vi "WriteStoreData.vi"(1 "Spots":T1[](array[typedef]) {"F2-Value overall" format="%.2f"; "tauerror" format="%.2f"; "Lifetime[ns]" format="%.2f"; "F2-Value TAC" format="%.2f"}, 2 "Enum":enum16{"Save", "Control"}(ring), 3 "Image Path":refnum<vi>) -> (0 "already x spots":i16)   [LabVIEW 2009]
uses:
  spotproperties.ctl
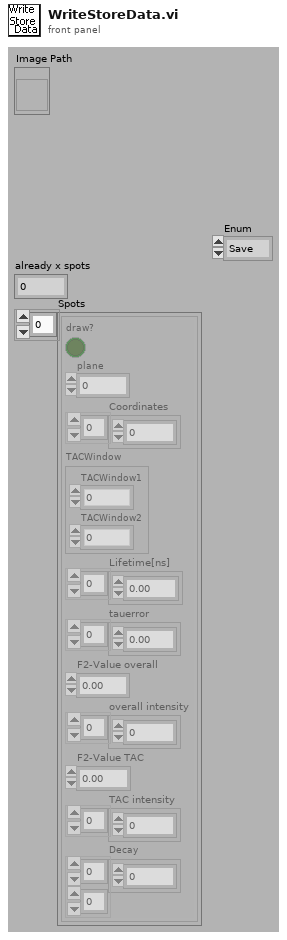
[diagram p1: front panel]
types:
  T1 = typedef "spotproperties.ctl" = cluster{"draw?":bool, "plane":u32, "Coordinates":i32[], "TACWindow":cluster{"TACWindow1":i32, "TACWindow2":i32}, "Lifetime[ns]":ext[], "tauerror":dbl[], "F2-Value overall":dbl, "overall intensity":u32[], "F2-Value TAC":dbl, "TAC intensity":u32[], "Decay":u32[][]}
  T2 = enum16{"Display", "change", "Get", "Set", "Set Ken"}
  T3 = enum16{"open", "open or create", "create or replace", "create", "open (read only)"}
  T4 = enum16{"read/write", "read-only", "write-only", "write-only (truncate)"}
  T5 = typedef "Settings.ctl" = cluster{"threshold":cluster{"max":u32, "min":u32}, "RGB or false color":bool, "16bit":bool, "log/lin axis":u16, "spotsize button":bool, "Pixelsize":u16, "autoscale x":bool, "autoscale y":bool, "correlation":bool, "ADC-Resolution":i32, "F2-lifetime":cluster{"display tau":bool, "display F2":bool, "Palette Number lifetime":enum32{"Gray", "Binary", "Gradient", "Rainbow", "Temperature"}, "Palette Number F2":enum32{"Gray", "Binary", "Gradient", "Rainbow", "Temperature"}, "max tau-Value":dbl, "min tau-Value":dbl, "max F2-Value":dbl, "min F2-Value":dbl}, "TAC-Window 1":u16, "TAC-Window 2":u16, "false color palette":cluster{"1":u32, "2":u32, "3":u32, "4":u32, "5":u32, "6":u32, "7":u32, "8":u32, "8 2":u32, "8 3":u32, "8 4":u32, "8 5":u32}, "rebinning":dbl}
  T6 = typedef "FIFOSettings_BH.ctt" = cluster{"Measurement":cluster{"Binning (ms)":sgl, "External Trigger Condition":u16, "Stop Condition:":u16, "Stop Count":dbl, "Buffer Size (Photons)":u16, "No of Channels":u16, "Ext Latch Delay":i16}, "ADC":cluster{"Module":u16, "ADC Resolution":i32, "Dither Range":i16, "Count Increment":i16, "Macro Time Clock":i16}, "SYNC":cluster{"SYNC ZC Level (mV)":sgl, "SYNC Freq Divider":i16, "SYNC Holdoff (ns)":sgl, "SYNC Threshold (mV)":sgl}, "TAC":cluster{"TAC Range (ns)":sgl, "TAC Gain":i16, "TAC Offset (%)":sgl, "TAC Limit Low (%)":sgl, "TAC Limit High (%)":sgl}, "CFD":cluster{"CFD Limit Low (mV)":sgl, "CFD Limit High (mV)":sgl, "CFD ZC Level (mV)":sgl, "CFD Holdoff (ns)":sgl}}
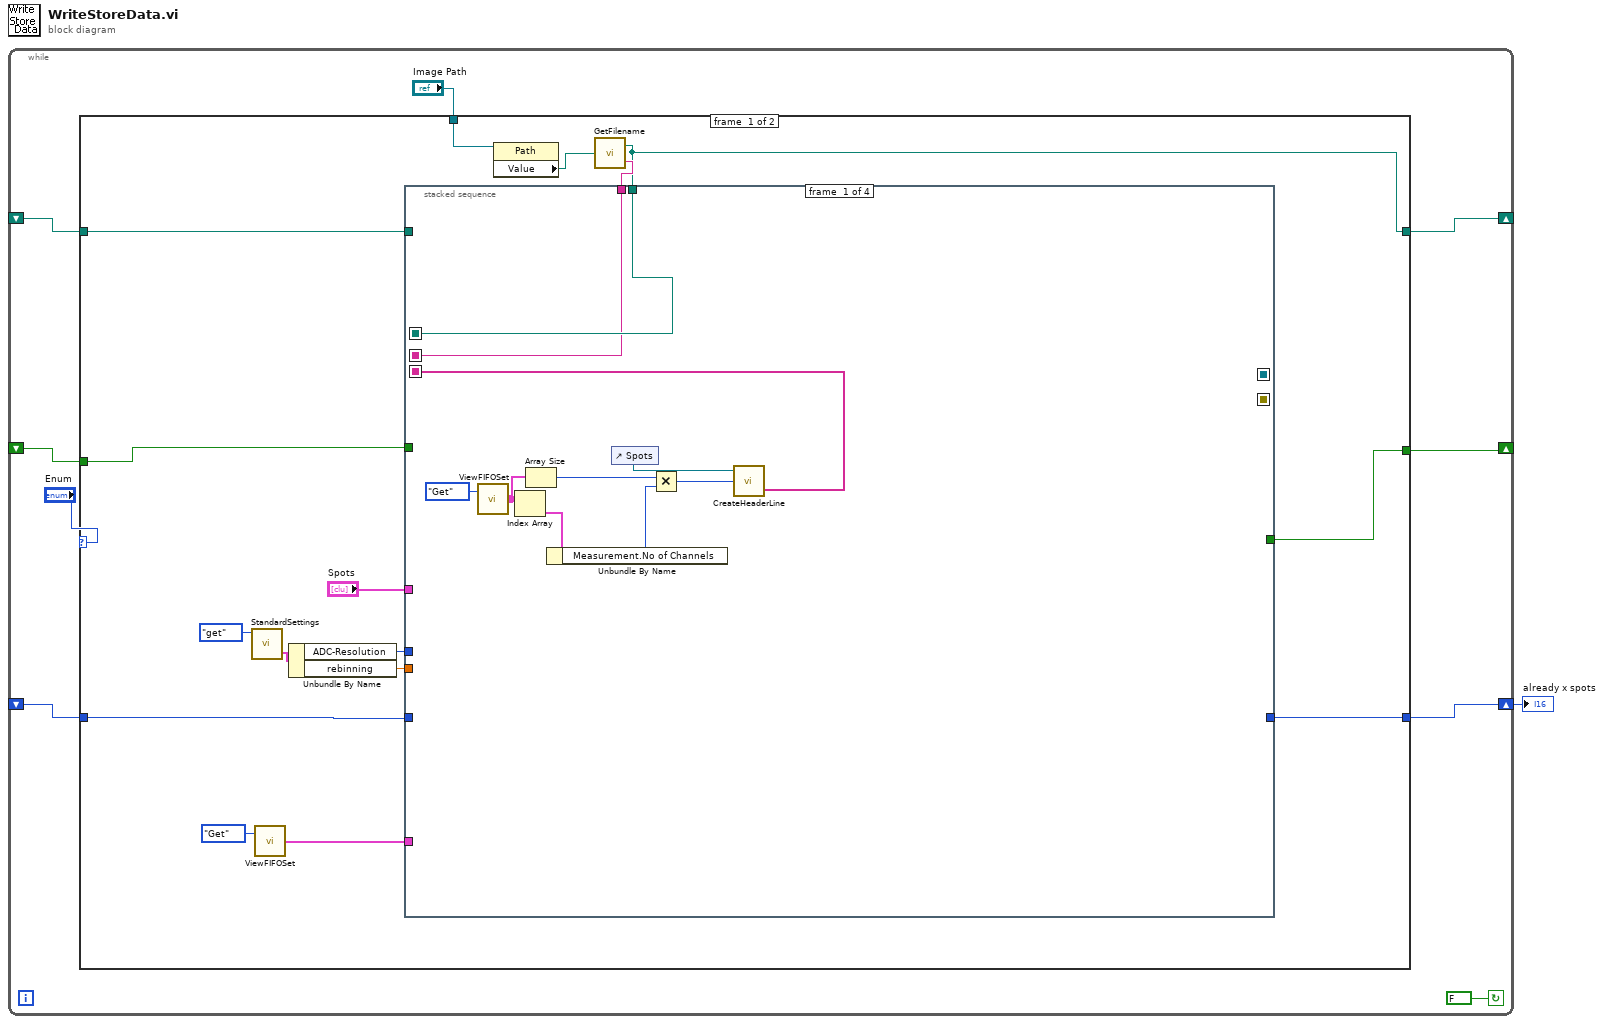
[diagram p0: block diagram]
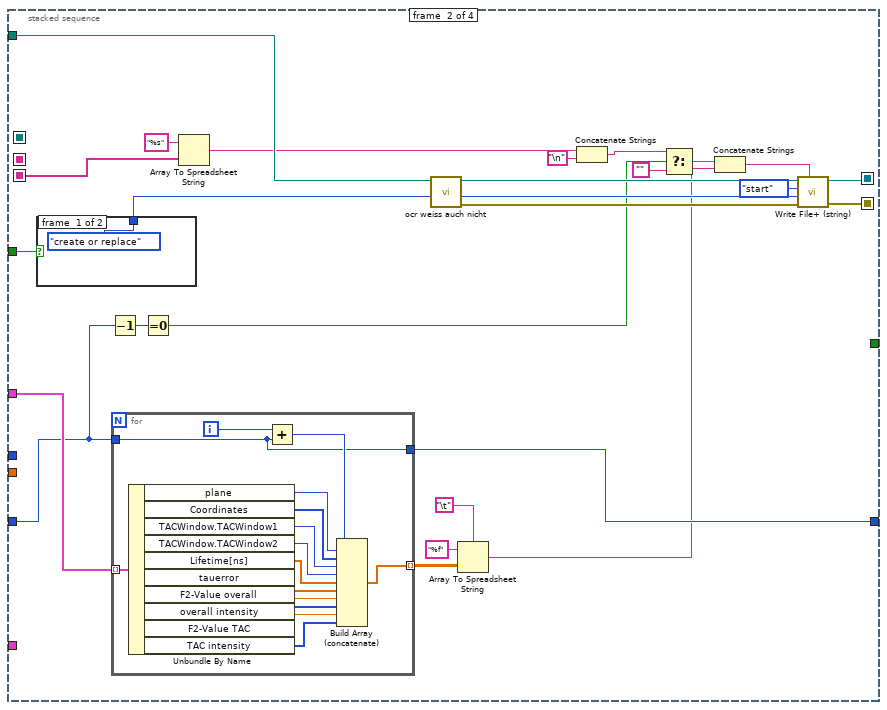
[diagram p2: hidden frame]
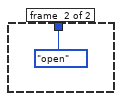
[diagram p3: hidden frame]
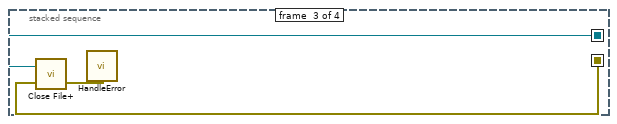
[diagram p4: hidden frame]
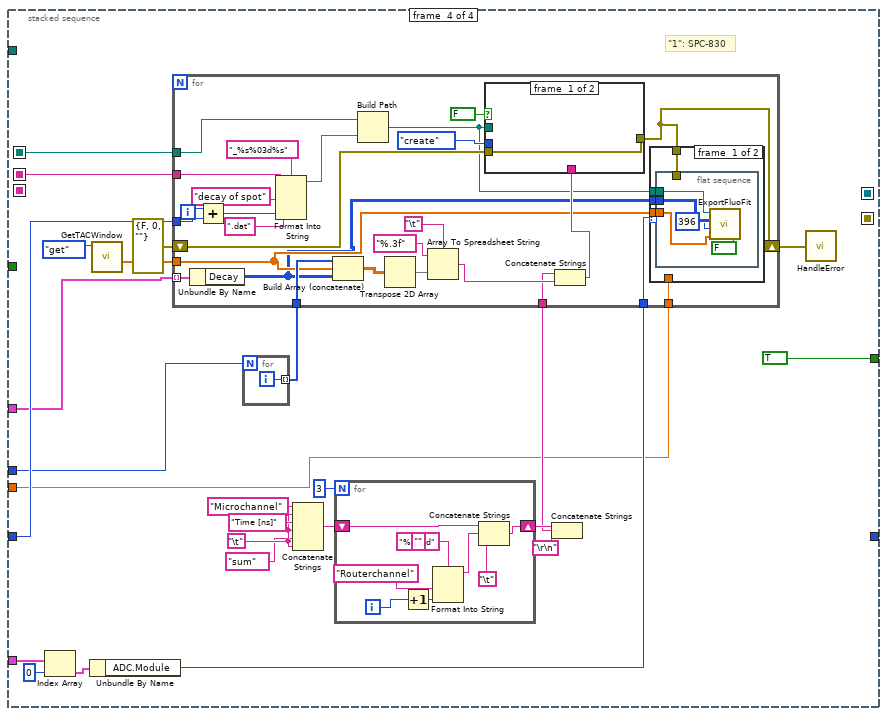
[diagram p5: hidden frame]
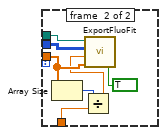
[diagram p6: hidden frame]
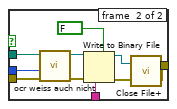
[diagram p7: hidden frame]
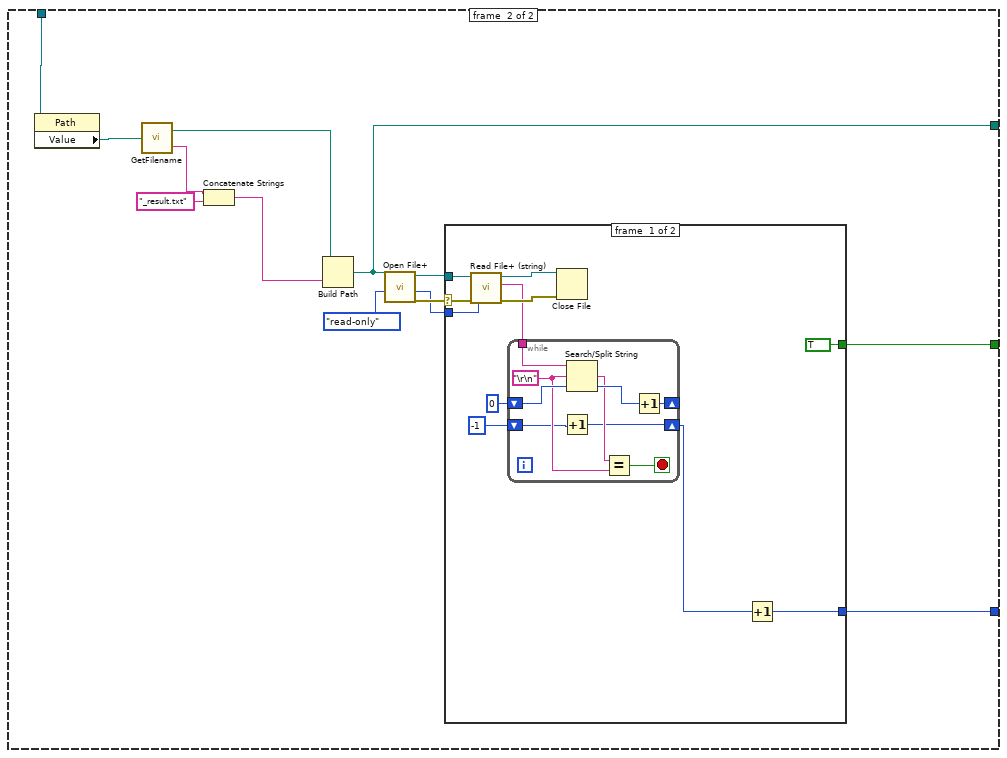
[diagram p8: hidden frame]
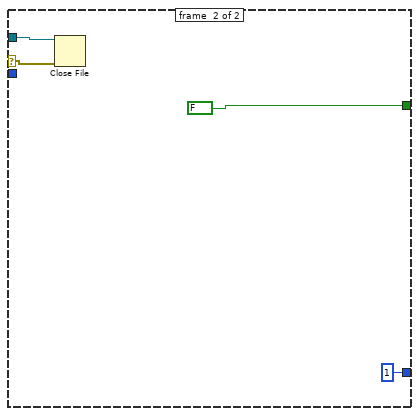
[diagram p9: hidden frame]
diagram:
  n1 = while {
    shift-right: [w8] -> _
    shift-left: _ -> [w7]
    shift-right: [w6] -> w1
    shift-left: _ -> [w5]
    shift-right: [w4] -> _
    shift-left: _ -> [w3]
    stop <- FALSE continue-if-true
    n2 = case shown="\"Save\", Default" "Enum" {
      tunnel: [w26 w183] -> w8
      tunnel: w7 -> [w25 _]
      tunnel: [w24 w171] -> w6
      tunnel: w5 -> [w18 _]
      tunnel: [w14 w173] -> w4
      tunnel: w3 -> [w23 _]
      tunnel: "Image Path" -> [w15 w172]
      frame #0 {
        n3 = call "StandardSettings.vi"("Enum"=enum16{"Load", "get", "Save", "set"}."get") -> ("StandardSettings"=w21:T5)  [unwired: 4 in]
        n4 = call "ViewFIFOSet.vi"("Enum"=T2."Get") -> ("FIFO Settings (Array)"=w12:T6[])  [unwired: 1 in]
        n5 = Unbundle By Name(w21) -> ("ADC-Resolution"=w20:i32, "rebinning"=w11:dbl)
        n6 = property class="Path"(reference=w15) -> ("Value"=w16:path)  [unwired: 1 in, 2 out]
        n7 = call "GetFilename.vi"("Value"=w16) -> ("base path"=w14:path, "name"=w17:string)
        n8 = stacked-sequence {
          seq-local: [w28 _ _ _] -> [_ _ _ w107]
          seq-local: [w27 _ _ _] -> [_ _ _ w95]
          seq-local: [w35 _ _ _] -> [_ w48 _ _]
          seq-local: [_ w61 _ _] -> [_ _ w82 _]
          seq-local: [_ w60 _ _] -> [_ _ w81 _]
          tunnel: "Spots" -> [_ w59 _ w92]
          tunnel: [_ _ _ TRUE] -> w26
          tunnel: w25 -> [_ w52 _ _]
          tunnel: [_ w51 _ _] -> w24
          tunnel: w18 -> [_ w44 _ w99]
          tunnel: w23 -> [_ w49 _ _]
          tunnel: w20 -> [_ _ _ w91]
          tunnel: w14 -> [w28 _ _ _]
          tunnel: w17 -> [w27 _ _ _]
          tunnel: w12 -> [_ _ _ w87]
          tunnel: w11 -> [_ _ _ w83]
          frame #0 {
            n9 = call "ViewFIFOSet.vi"("Enum"=T2."Get") -> ("FIFO Settings (Array)"=w30:T6[])  [unwired: 1 in]
            n10 = Index Array(array=w30) -> (element=w33:T6)  [unwired: 1 in]
            n11 = Array Size(array=w30) -> (size(s)=w31:i32)
            n12 = Unbundle By Name(w33) -> ("Measurement.No of Channels"=w32:u16)
            n13 = control-ref of="Spots"() -> (w36:refnum<vi>)
            n14 = Multiply(x=w31, y=w32) -> (x*y=w29:i32)
            n15 = call "CreateHeaderLine.vi"("No of channels"=w29, "Spots 3"=w36) -> ("Headline array"=w35:string[])  [unwired: 2 in]
          }
          frame #1 {
            n16 = case shown="True" w52 {
              tunnel: [T3."create or replace" ("function (open:0)") T3."open" ("function (open:0)")] -> w62
              frame #0 {
              }
              frame #1 {
              }
            }
            n17 = Decrement(x=w44) -> (x-1=w45:i16)
            n18 = for {
              tunnel: w59 -> [w79] mode=indexing
              tunnel: [w78] -> w58 mode=indexing
              tunnel: [w75] -> w51
              tunnel: w44 -> [w75]
              i -> [w77]
              n19 = Unbundle By Name(w79) -> ("plane"=w74:u32, "Coordinates"=w73:i32[], "TACWindow.TACWindow1"=w72:i32, "TACWindow.TACWindow2"=w71:i32, "Lifetime[ns]"=w70:ext[], "tauerror"=w69:dbl[], "F2-Value overall"=w68:dbl, "overall intensity"=w67:u32[], "F2-Value TAC"=w66:dbl, "TAC intensity"=w65:u32[])
              n20 = Add(x=w77, y=w75) -> (x+y=w76:i32)
              n21 = Build Array (concatenate)(w76, w74, w73, w72, w71, w70, w69, w68, w67, w66, w65) -> (w78:ext[])
            }
            n22 = Equal To 0?(x=w45) -> (x = 0?=w43:bool)
            n23 = Array To Spreadsheet String(array=w48, 3:"%s" ("format string")) -> (spreadsheet string=w46:string)  [unwired: 1 in]
            n24 = call "ocr weiss auch nicht.vi"("function (open:0)"=w62, "file path"=w49) -> ("error out"=w55:errorcluster, "file size (bytes)"=w53:i32, "refnum"=w56:refnum<file>)  [unwired: 6 in, 1 out]
            n25 = Array To Spreadsheet String(delimiter (Tab)="\t", array=w58, 3:"%f" ("format string")) -> (spreadsheet string=w39:string)
            n26 = Concatenate Strings(w46, "\n") -> (w42:string)
            n27 = Select(t=w42, s=w43, f="") -> (s? t:f=w40:string)
            n28 = Concatenate Strings(w40, w39) -> (w38:string)
            n29 = call "Write File+ (string).vi"("string"=w38, "error in (no error)"=w55, "pos offset (bytes:0)"=w53, "pos mode (rel. to end:1)"=enum16{"start", "end", "current"}."start", "refnum"=w56) -> ("error out"=w60:errorcluster, "dup refnum"=w61:refnum<file>)  [unwired: 2 in, 1 out]
          }
          frame #2 {
            n30 = call "Close File+.vi"("error in (no error)"=w81, "refnum"=w82) -> ("error out"=w80:errorcluster)  [unwired: 3 in, 2 out]
            n31 = call "HandleError.vi"("error in (no error)"=w80) -> ()
          }
          frame #3 {
            w94 = "\t"
            # "\"1\": SPC-830"
            n32 = Index Array(array=w87, index=0) -> (element=w85:T6)
            n33 = Unbundle By Name(w85) -> ("ADC.Module"=w84:u16)
            n34 = call "GetTACWindow.vi"("Enum"=enum16{"ini", "get", "quick"}."get") -> ("x-values"=w88:dbl[])  [unwired: 1 in, 8 out]
            n35 = for {
              N: w91 -> [_]
              tunnel: [w108] -> w97 mode=indexing
              i -> [w108]
            }
            n36 = Concatenate Strings("Microchannel" ("string"), w94, "Time [ns]" ("string"), w94, "sum" ("string"), w94) -> (w101:string)
            n37 = for {
              N: 3 -> [_]
              shift-right: [w116] -> w105
              shift-left: w101 -> [w115]
              i -> [w113]
              (unwired) "%s %d" ("format string")
              n38 = Increment(x=w113) -> (x+1=w112:i32)
              n39 = Format Into String(format string="", "Routerchannel", w112) -> (resulting string=w110:string)  [unwired: 2 in, 1 out]
              n40 = Concatenate Strings(w115, w110, "\t") -> (w116:string)
            }
            n41 = Concatenate Strings(w105, "\r\n") -> (w104:string)
            n42 = for {
              tunnel: w92 -> [w143] mode=indexing
              tunnel: w107 -> [w142]
              tunnel: w88 -> [w123]
              shift-right: [w121] -> w89
              shift-left: errorcluster {"status"=FALSE, "code"=0, "source"=""} ("error out") -> [w137]
              tunnel: w104 -> [w134]
              tunnel: w99 -> [w129]
              tunnel: w95 -> [w124]
              tunnel: w97 -> [w125]
              tunnel: w84 -> [w118]
              tunnel: w83 -> [w117]
              i -> [w130]
              n43 = Unbundle By Name(w143) -> ("Decay"=w119:u32[][])
              n44 = Add(x=w130, y=w129) -> (x+y=w128:i32)
              n45 = Format Into String(format string="_%s%03d%s", initial string=w124, "decay of spot", w128, ".dat" ("replace string (\"\")")) -> (resulting string=w132:string)  [unwired: 1 in, 1 out]
              n46 = Build Array (concatenate)(w125, w123, w119) -> (w140:dbl[][])
              n47 = Build Path(base path=w142, name or relative path=w132) -> (appended path=w122:path)
              n48 = Transpose 2D Array(2D array=w140) -> (transposed array=w139:dbl[][])
              n49 = Array To Spreadsheet String(delimiter (Tab)="\t", array=w139, 3:"%.3f" ("format string")) -> (spreadsheet string=w136:string)
              n50 = Concatenate Strings(w134, w136) -> (w135:string)
              n51 = case shown="False" FALSE {
                tunnel: w137 -> [w160 w166]
                tunnel: w135 -> [_ w165]
                tunnel: T3."create" ("function (open:0)") -> [_ w164]
                tunnel: w122 -> [_ w163]
                tunnel: [w160 w162] -> w121
                frame #0 {
                }
                frame #1 {
                  n52 = call "ocr weiss auch nicht.vi"("error in (no error)"=w166, "function (open:0)"=w164, "file path"=w163) -> ("error out"=w167:errorcluster, "refnum"=w168:refnum<file>)  [unwired: 5 in, 2 out]
                  n53 = Write to Binary File(file (use dialog)=w168, data=w165, error in=w167, 5:FALSE ("prepend array or string size? (T)")) -> (refnum out=w169:refnum<file>, error out=w170:errorcluster)  [unwired: 2 in, 1 out]
                  n54 = call "Close File+.vi"("error in (no error)"=w170, "refnum"=w169) -> ("error out"=w162:errorcluster)  [unwired: 3 in, 2 out]
                }
              }
              n55 = case shown="1" w118 {
                tunnel: w123 -> [w147 w156]
                tunnel: w122 -> [w146 w159]
                tunnel: w121 -> [w145 _]
                tunnel: w119 -> [w144 w158]
                tunnel: w117 -> [_ w154]
                frame #0 {
                  n56 = flat-sequence {
                    tunnel: w147 -> [w149]
                    tunnel: w146 -> [w150]
                    tunnel: w145 -> [_]
                    tunnel: w144 -> [w152]
                    frame #0 {
                      n57 = call "ExportFluoFit.vi"("from end?"=FALSE, "time in"=w149, "# of lines"=396, "lifetimes"=w152, "Lifetime Export Path (ASCII-File)"=w150) -> ()  [unwired: 2 in]
                    }
                  }
                }
                frame #1 {
                  n58 = Array Size(array=w156) -> (size(s)=w155:i32)
                  n59 = Divide(x=w155, y=w154) -> (x/y=w153:dbl)
                  n60 = call "ExportFluoFit.vi"("from end?"=TRUE, "time in"=w156, "# of lines"=w153, "lifetimes"=w158, "Lifetime Export Path (ASCII-File)"=w159) -> ()  [unwired: 2 in]
                }
              }
            }
            n61 = call "HandleError.vi"("error in (no error)"=w89) -> ()
          }
        }
      }
      frame #1 {
        n62 = property class="Path"(reference=w172) -> ("Value"=w178:path)  [unwired: 1 in, 2 out]
        n63 = call "GetFilename.vi"("Value"=w178) -> ("base path"=w176:path, "name"=w177:string)
        n64 = Concatenate Strings(w177, "_result.txt" ("string")) -> (w174:string)
        n65 = Build Path(base path=w176, name or relative path=w174) -> (appended path=w173:path)
        n66 = call "Open File+.vi"("open mode (read-only:1)"=T4."read-only", "file path (\" \")"=w173) -> ("error out"=w180:errorcluster, "file size (bytes)"=w179:i32, "refnum"=w181:refnum<file>)  [unwired: 6 in, 1 out]
        n67 = case shown="No Error" w180 {
          selector: w180 -> [w192 w204]
          tunnel: w181 -> [w193 w205]
          tunnel: [TRUE FALSE] -> w183
          tunnel: [w184 i16 1] -> w171
          tunnel: w179 -> [w186 _]
          frame #0 {
            n68 = call "Read File+ (string).vi"("count"=w186, "error in (no error)"=w192, "refnum"=w193) -> ("error out"=w190:errorcluster, "string"=w189:string, "dup refnum"=w191:refnum<file>)  [unwired: 4 in, 2 out]
            n69 = while {
              shift-right: [w195] -> _
              shift-left: 0 ("offset of match") -> [w201]
              shift-right: [w196] -> w185
              shift-left: i16 -1 -> [w197]
              tunnel: w189 -> [w203]
              stop <- w198 stop-if-true
              w199 = "\r\n"
              n70 = Increment(x=w197) -> (x+1=w196:i16)
              n71 = Search/Split String(string=w203, search string/char (-)=w199, offset (0)=w201) -> (match + rest of string=w200:string, offset of match=w202:i32)  [unwired: 1 out]
              n72 = Equal?(x=w200, y=w199) -> (x = y?=w198:bool)
              n73 = Increment(x=w202) -> (x+1=w195:i32)
            }
            n74 = Close File(refnum=w191, error in=w190) -> ()  [unwired: 2 out]
            n75 = Increment(x=w185) -> (x+1=w184:i16)
          }
          frame #1 {
            n76 = Close File(refnum=w205, error in=w204) -> ()  [unwired: 2 out]
          }
        }
      }
    }
  }
  "already x spots" <- w1
